vi "MPM_Get_Wavelength.vi"(8 "error in (no error)":errorcluster, 11 ".NET Reference in":refnum<k24>) -> (0 "error out":errorcluster, 2 "wave out":dbl, 3 "Reference out":refnum<k24>)   [LabVIEW 2017]
doc: "get setting wavelength(nm)"
uses:
  D:/test/FULLband-sts/Fullband_Sample/DLL/InstrumentDLL.dll
  DLL/InstrumentDLL.dll
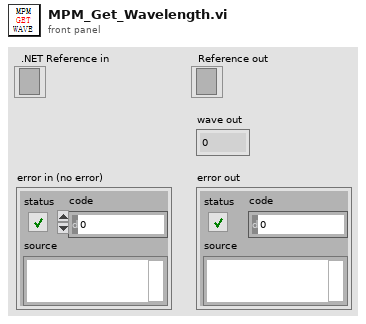
[diagram p1: front panel]
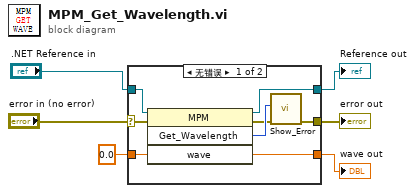
[diagram p0: block diagram]
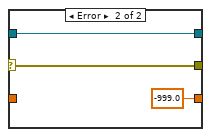
[diagram p2: hidden frame]
diagram:
  n1 = case shown="无错误" "error in (no error)" {
    selector: "error in (no error)" -> [w7 w17]
    tunnel: [w14 w16] -> w6
    tunnel: [w13 -999.0 ("wave")] -> w5
    tunnel: ".NET Reference in" -> [w12 w16]
    tunnel: 0.0 ("wave") -> [w11 _]
    tunnel: [w8 w17] -> w2
    frame No Error {
      n2 = invoke on="调用节点" class="MPM" method="Get_Wavelength"(reference=w12, error in=w7, "wave"=w11) -> (reference out=w14:refnum<k24>, error out=w9:errorcluster, "Get_Wavelength"=w10:i32, "wave"=w13:dbl)  [unwired: 1 in]
      n3 = call "Show_Error.vi"("error in (no error)"=w9, "Error"=w10) -> ("error out"=w8:errorcluster)  [unwired: 9 in]
    }
    frame Error {
    }
  }
  "Reference out" <- w6
  "wave out" <- w5
  "error out" <- w2
